vi "Move.vi"(5 "Movement Type (0: relative)":u16(ring) items=["relative", "absolute"], 6 "error in (no error)":errorcluster, 8 "XYZ In":dbl[](array[numeric]), 9 "VISA Refnum in":refnum<visa-resource-name>) -> (0 "error out":errorcluster, 3 "VISA Refnum out":refnum<visa-resource-name>)   [LabVIEW 2018, in "Stage Actor.lvlib"]
uses:
  Stage Actor.lvlib
  <instrlib>/Zaber A Series/Zaber A Series.lvlib
panel:
  in  "Z Device and Axis (03) in":string="03"
  in  "Z-Axis Microstep Size (0) in":dbl=0.047625
  in  "Y Device and Axis (02) in":string="02"
  in  "Y-Axis Microstep Size (0) in":dbl=0.047625
  in  "X Device and Axis (01) 3":string="01"
  in  "X-Axis Microstep Size (0) 3":dbl=0.047625
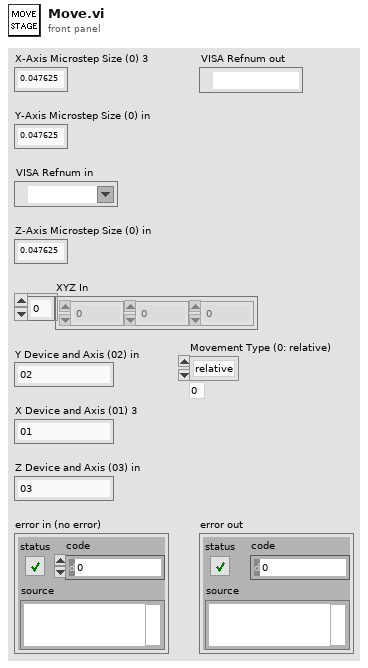
[diagram p1: front panel]
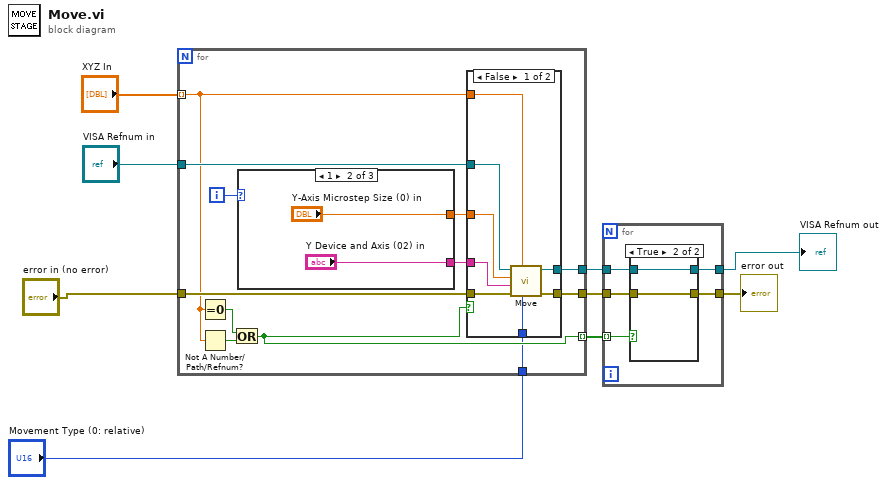
[diagram p0: block diagram]
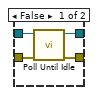
[diagram p2: hidden frame]
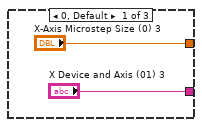
[diagram p3: hidden frame]
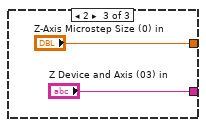
[diagram p4: hidden frame]
diagram:
  n1 = for {
    tunnel: "XYZ In" -> [w14] mode=indexing
    tunnel: "VISA Refnum in" -> [w19]
    tunnel: "error in (no error)" -> [w18]
    tunnel: [w13] -> w8
    tunnel: [w12] -> w7
    tunnel: [w11] -> w3 mode=indexing
    tunnel: "Movement Type (0: relative)" -> [w10]
    i -> [w17]
    n2 = Equal To 0?(x=w14) -> (x = 0?=w21:bool)
    n3 = Not A Number/Path/Refnum?(number/path/refnum=w14) -> (NaN/Path/Refnum?=w20:bool)
    n4 = Or(x=w21, y=w20) -> (x .or. y?=w11:bool)
    n5 = case shown="1" w17 {
      tunnel: ["X-Axis Microstep Size (0) 3" "Y-Axis Microstep Size (0) in" "Z-Axis Microstep Size (0) in"] -> w16
      tunnel: ["X Device and Axis (01) 3" "Y Device and Axis (02) in" "Z Device and Axis (03) in"] -> w15
      frame 0, Default {
      }
      frame 1 {
      }
      frame 2 {
      }
    }
    n6 = case shown="False" w11 {
      tunnel: w19 -> [w35 w37]
      tunnel: w15 -> [w34 _]
      tunnel: w18 -> [w33 w36]
      tunnel: w16 -> [w32 _]
      tunnel: w14 -> [w31 _]
      tunnel: [w30 w37] -> w13
      tunnel: [w29 w36] -> w12
      tunnel: w10 -> [w28 _]
      frame False {
        n7 = call <instrlib>:"Move.vi"("Movement Type (0: relative)"=w28, "Move Distance (0)"=w31, "error in (no error)"=w33, "Device and Axis"=w34, "Microstep Size (0)"=w32, "VISA resource name"=w35) -> ("error out"=w29:errorcluster, "VISA resource name out"=w30:refnum<visa-resource-name>)  [unwired: 4 in]
      }
      frame True {
      }
    }
  }
  n8 = for {
    tunnel: w8 -> [w42]
    tunnel: w7 -> [w41]
    tunnel: [w40] -> w5
    tunnel: [w39] -> w6
    tunnel: w3 -> [w38] mode=indexing
    n9 = case shown="True" w38 {
      tunnel: w42 -> [w46 w48]
      tunnel: w41 -> [w45 w47]
      tunnel: [w44 w48] -> w40
      tunnel: [w43 w47] -> w39
      frame False {
        n10 = call <instrlib>:"Poll Until Idle.vi"("error in (no error)"=w45, "VISA resource name"=w46) -> ("error out"=w43:errorcluster, "VISA resource name out"=w44:refnum<visa-resource-name>)  [unwired: 8 in]
      }
      frame True {
      }
    }
  }
  "error out" <- w6
  "VISA Refnum out" <- w5
